vi "SecurityOffFGV.vi"(8 "error in":errorcluster, 10 "Set_Get":enum16{"Set", "Get"}(ring)=enum."Get", 11 "Value":bool=TRUE) -> (0 "error out":errorcluster, 3 "Get":bool)   [LabVIEW 2010]
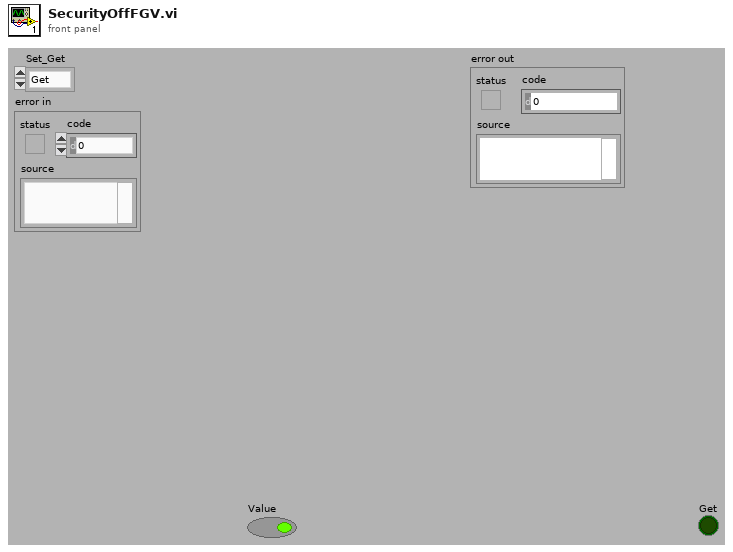
[diagram p1: front panel]
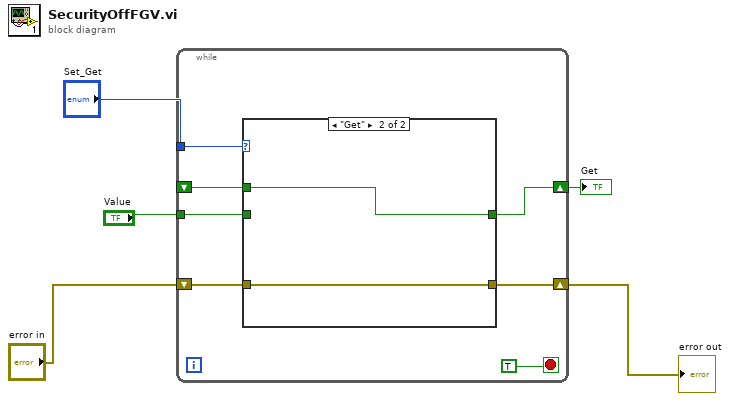
[diagram p0: block diagram]
diagram:
  n1 = while {
    tunnel: "Set_Get" -> [w12]
    tunnel: "Value" -> [w11]
    shift-right: [w10] -> w4
    shift-left: _ -> [w9]
    shift-right: [w6] -> w1
    shift-left: "error in" -> [w7]
    stop <- TRUE stop-if-true
    n2 = case shown="\"Get\"" w12 {
      tunnel: w11 -> [w14 _]
      tunnel: [w14 w16] -> w10
      tunnel: w9 -> [_ w16]
      tunnel: w7 -> [w13 w15]
      tunnel: [w13 w15] -> w6
      frame "Set", Default {
      }
      frame "Get" {
      }
    }
  }
  "Get" <- w4
  "error out" <- w1
